vi "Single Lockin.vi"() -> ()   [LabVIEW 2013]
uses:
  NILockin/Lockin Configuration.ctl
  <vilib>/measure/NI_MABase.lvlib
panel:
  out "Frequency Detected":dbl=102.40333431899356 format="%.2f"
  in  "stop":bool
  out "Amplitude":dbl[](graph)
  in  "Lock-in Configuration":T1={"Type"=enum."FIR", "TC (s)"=1.0, "Filter \nRolloff"=enum."20 dB", "Order"=1} {"Order" min=1 step=1; "TC (s)" format="%.3p"}
  in  "Reference Frequency":dbl=1000.0 format="%0.2p"
  in  "Noise Level":dbl=1.0 format="%.2p"
  in  "Amplitude":dbl=1.0 format="%0.2p"
  in  "Frequency":dbl=1000.0 format="%0.2p"
  out "Reference":waveform(dbl)(graph)
  out "Signal + Noise":waveform(dbl)(graph)
  out "Noise":waveform(dbl)(graph)
  out "Signal":waveform(dbl)(graph)
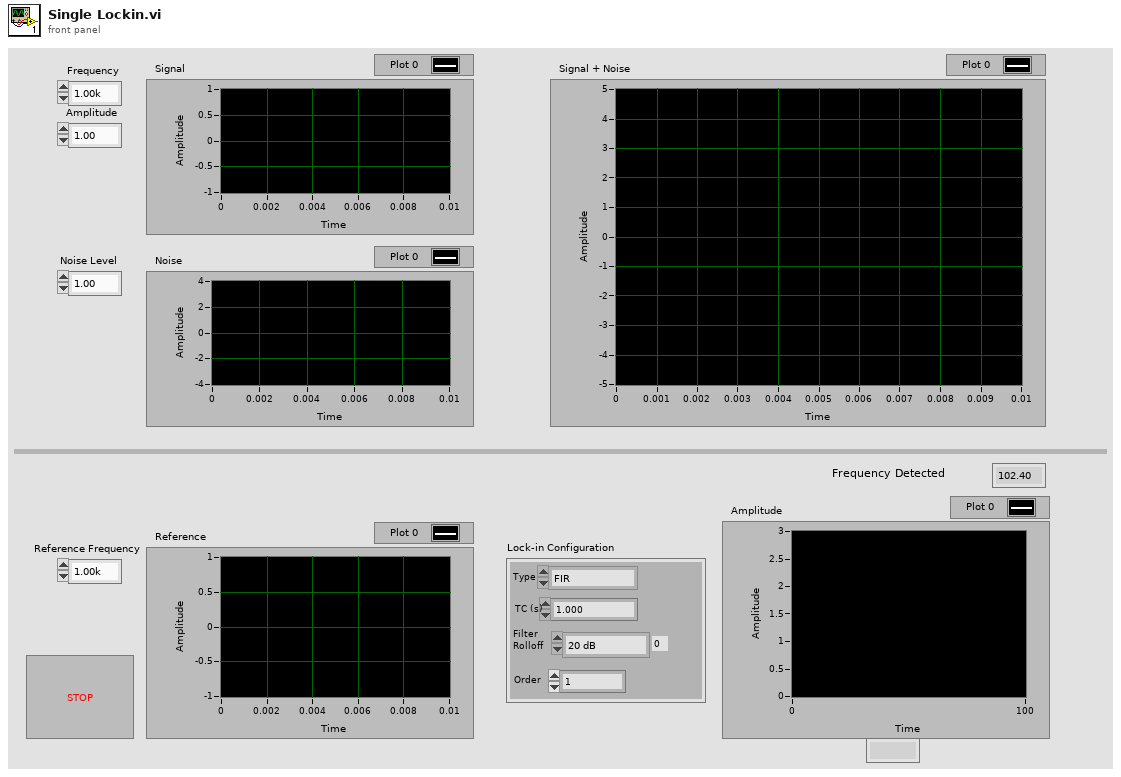
[diagram p1: front panel]
types:
  T1 = typedef "Lockin Configuration.ctl" = cluster{"Type":enum16{"IIR (2-dig)", "IIR (5-dig)", "FIR", "FIR (ENBW)", "FIR (Sync)"}, "TC (s)":dbl, "Filter \nRolloff":enum16{"20 dB", "40 dB", "60 dB", "80 dB", "100 dB", "120 dB", "140 dB", "160 dB", "180 dB", "200 dB"}, "Order":u32}
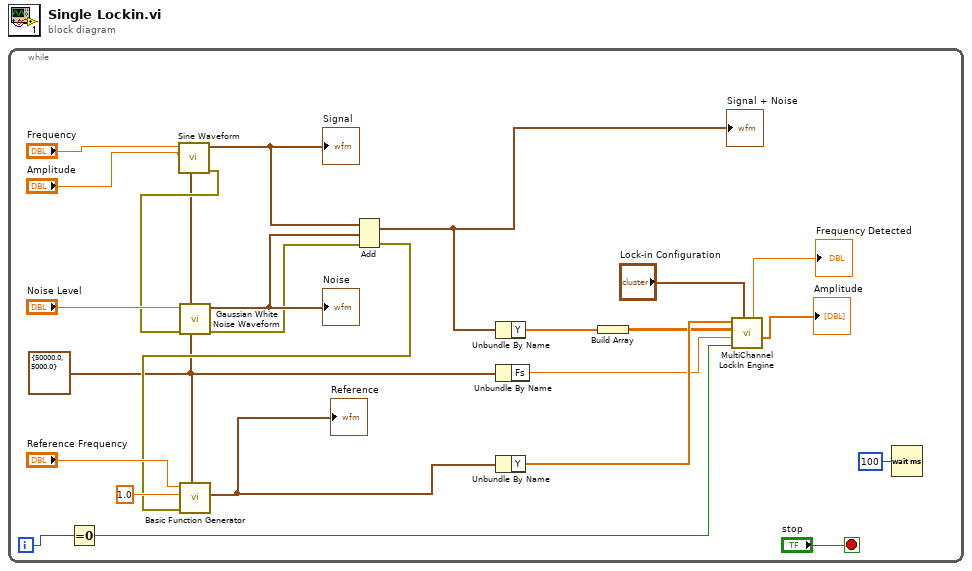
[diagram p0: block diagram]
diagram:
  n1 = while {
    i -> [w6]
    stop <- "stop" stop-if-true
    w8 = cluster{"Fs":dbl, "#s":dbl} {"Fs"=50000.0, "#s"=5000.0} ("sampling info")
    n2 = Equal To 0?(x=w6) -> (x = 0?=w5:bool)
    n3 = call <vilib>:"Sine Waveform.vi"("sampling info"=w8, "amplitude"="Amplitude", "frequency"="Frequency") -> ("error out"=w16:errorcluster, "signal out"=w15:waveform(dbl))  [unwired: 7 in]
    "Signal" <- w15
    n4 = call <vilib>:"Gaussian White Noise Waveform.vi"("sampling info"=w8, "error in (no error)"=w16, "standard deviation"="Noise Level") -> ("error out"=w22:errorcluster, "signal out"=w24:waveform(dbl))  [unwired: 7 in]
    "Noise" <- w24
    n5 = Add(1:w24, 2:w15, 4:w22) -> (0:w13:waveform(dbl), 3:w19:errorcluster)
    "Signal + Noise" <- w13
    n6 = call <vilib>:"Basic Function Generator.vi"("sampling info"=w8, "error in (no error)"=w19, "amplitude"=1.0, "frequency"="Reference Frequency") -> ("signal out"=w12:waveform(dbl))  [unwired: 5 in, 2 out]
    "Reference" <- w12
    n7 = Unbundle By Name(w13) -> ("Y"=w9:dbl[])
    n8 = Unbundle By Name(w8) -> ("Fs"=w7:dbl)
    n9 = Unbundle By Name(w12) -> ("Y"=w11:dbl[])
    n10 = Build Array(w9) -> (w10:dbl[][])
    n11 = call "MultiChannel LockIn Engine.vi"("Lock-in Configuration"="Lock-in Configuration", "Apply Change"=w5, "Sampling Rate"=w7, "Signals"=w10, "Reference Signal"=w11) -> ("R"=→"Amplitude":dbl[], "Frequency"=→"Frequency Detected":dbl)  [unwired: 1 in, 4 out]
    n12 = Wait (ms)(milliseconds to wait=u32 100) -> ()  [unwired: 1 out]
  }
